vi "PH_ImageOperator.Indicate Beam Analysis.vi"(0 "i ref in":refnum<vi>, 5 "error in (no error)":errorcluster) -> (14 "i ref out":refnum<vi>, 19 "error out":errorcluster)   [LabVIEW 2014, in "PH_ImageOperator.lvlib"]
doc: "This VI sets all GUI elements related to beam anaysis."
uses:
  PH_ImageOperator.lvlib
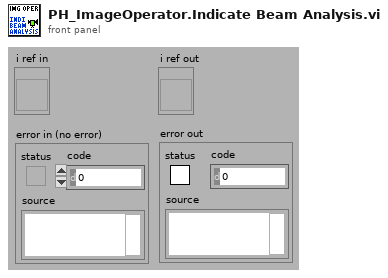
[diagram p1: front panel]
types:
  T1 = typedef "PH_ImageOperator.lvlib/PH_ImageOperator.i attribute.ctl" = cluster{"GUI Refs":cluster{"Delete":refnum<vi>, "Calibration status":refnum<vi>, "BI subtracted":refnum<vi>, "calc Energy":refnum<vi>, "Energy: expected value":refnum<vi>, "Energy: Tolerance":refnum<vi>, "Energy calculated":refnum<vi>, "Energy":refnum<vi>, "calc Beam Anal":refnum<vi>, "Maj Diam 1/esquare":refnum<vi>, "Min Diam 1/esquare":refnum<vi>, "Azi Angle":refnum<vi>, "Min/Maj Diam esquare":refnum<vi>, "Beam analysed":refnum<vi>, "CoG - x":refnum<vi>, "CoG - y":refnum<vi>, "BA: Method":refnum<vi>, "BA: Steps":refnum<vi>, "BA: Factor":refnum<vi>, "calc Traces":refnum<vi>, "Traces: Fit Gauss":refnum<vi>, "Traces calculated":refnum<vi>, "Maj FWHM":refnum<vi>, "Min FWHM":refnum<vi>, "Major Trace":refnum<vi>, "Minor Trace":refnum<vi>, "Maj Fit Order":refnum<vi>, "Min Fit Order":refnum<vi>, "Position calculated":refnum<vi>, "Position":refnum<vi>, "Type":refnum<vi>, "Center":refnum<vi>, "exp - X":refnum<vi>, "exp - Y":refnum<vi>, "Tolerance":refnum<vi>, "f":refnum<vi>, "M":refnum<vi>, "D":refnum<vi>, "q":refnum<vi>, "Dummy Method":refnum<vi>, "Dummy Type":refnum<vi>, "Global On":refnum<vi>, "Traces: No offset":refnum<vi>, "Maj 99%":refnum<vi>, "Min 99%":refnum<vi>, "GUI FF Image":refnum<vi>, "calc Fill Factor":refnum<vi>, "FF calculated":refnum<vi>, "Fill Factor: Filter?":refnum<vi>, "FF: Damage Threshold":refnum<vi>, "FF: Threshold":refnum<vi>, "FF: max allow. Energy":refnum<vi>, "FF: Fillfactor":refnum<vi>, "Calibration data":refnum<vi>}, "List of GUIs":string[], "Calibration":cluster{"Status":T2, "Calibration data":T3, "Calibration Data File":path}, "Final Image":cluster{"BI Subtraction Failure":bool}, "Energy":cluster{"on":bool, "expected value [mJ]":dbl, "Tolerance [%]":dbl, "State":T2, "Energy [mJ]":dbl, "Unit":string, "calculated @":timestamp}, "Beam Analysis":cluster{"on":bool, "Data":T4, "Method":bool, "Steps":i32, "Factor":i32, "ROI":cluster{"Left":i32, "Top":i32, "Right":i32, "Bottom":i32}, "analysed @":timestamp}, "Trace Analysis":cluster{"on":bool, "Fit on":bool, "Maj FWHM":dbl, "Min FWHM":dbl, "Maj Fit Order":i32, "Min Fit Order":i32, "No Offset":bool, "Maj 99%":dbl, "Min 99%":dbl, "Traces":cluster{"XScaleName":string, "Y Scale Minimum":sgl, "Y Scale Maximum":sgl, "X Scale Minimum":sgl, "X Scale Maximum":sgl, "Traces":cluster{"Index":sgl[], "Trace":dbl[]}[]}[], "analysed @":timestamp}, "Position Analysis":cluster{"on":bool, "exp - X":i32, "exp - Y":i32, "focal length [mm]":dbl, "Magnification":dbl, "Delta":dbl, "Theta":dbl, "Tolerance":dbl, "Type":bool, "analysed @":timestamp}, "Fill Factor":cluster{"on":bool, "Filter on?":bool, "Threshold":dbl, "Damage Threshold [J/cm²]":dbl, "Fillfactor":dbl, "Max. allowed Energy [J]":dbl, "calculated @":timestamp}, "Statistician Service ID":i32, "Images":cluster{"Background":T5, "OP":T5, "GUI":T5, "BA: ROI":T5, "Trace: Turn":T5, "FF: Main":T5, "FF: Help":T5, "PSDB: BG":T5, "PSDB: OP":T5, "PSDB: FF":T5}}
  T2 = typedef "PH_StatusHandler.lvlib/PH_StatusHandler.Status.ctl" = i16
  T3 = typedef "PH_ImageCalibrator.lvlib/PH_ImageCalibrator.Calibration Data.ctl" = cluster{"Date":string, "Time":string, "Cam Settings":cluster{"Cam ID":string, "Gain":dbl, "Brightness":dbl, "Shutter":dbl, "Cam Error":bool, "Mode":i32}, "Background Image":cluster{"Image":dbl[][], "Image Error":bool}, "Linear Calibration":cluster{"Calibration Factor":dbl, "not mm or mrad":bool}, "Energy Calibration":cluster{"Calibration Factor":dbl, "no mJ":bool}}
  T4 = typedef "PH_ImageOperator.lvlib/PH_ImageOperator.Beam Analysis Data.ctl" = cluster{"CoG-x":sgl, "CoG-y":sgl, "Maj Dim":dbl, "Min Dim":dbl, "Ellipticity":dbl, "Azimuth Angle [rad]":dbl, "Azi Angle rel to Maj?":bool}
  T5 = typedef "IMAQ Image.ctl" = refnum<image>
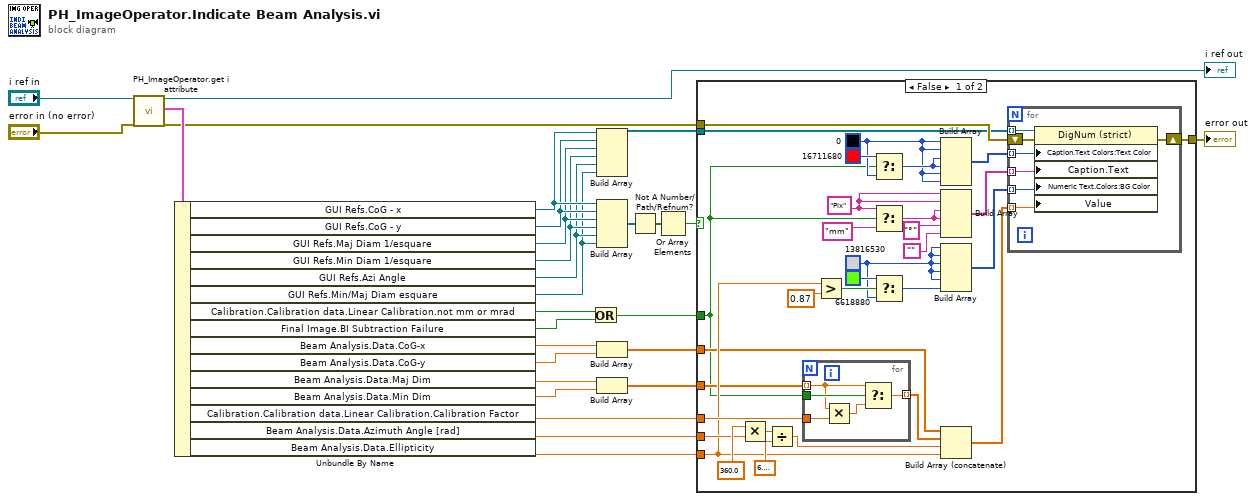
[diagram p0: block diagram]
diagram:
  n1 = call "PH_ImageOperator.get i attribute.vi"("i ref in"="i ref in", "error in (no error)"="error in (no error)") -> ("i ref out"=→"i ref out":refnum<vi>, "i attribute"=w25:T1, "error out"=w19:errorcluster)  [unwired: 15 in]
  n2 = Unbundle By Name(w25) -> ("GUI Refs.CoG - x"=w18:refnum<vi>, "GUI Refs.CoG - y"=w17:refnum<vi>, "GUI Refs.Maj Diam 1/esquare"=w16:refnum<vi>, "GUI Refs.Min Diam 1/esquare"=w15:refnum<vi>, "GUI Refs.Azi Angle"=w14:refnum<vi>, "GUI Refs.Min/Maj Diam esquare"=w13:refnum<vi>, "Calibration.Calibration data.Linear Calibration.not mm or mrad"=w3:bool, "Final Image.BI Subtraction Failure"=w2:bool, "Beam Analysis.Data.CoG-x"=w6:sgl, "Beam Analysis.Data.CoG-y"=w5:sgl, "Beam Analysis.Data.Maj Dim"=w10:dbl, "Beam Analysis.Data.Min Dim"=w11:dbl, "Calibration.Calibration data.Linear Calibration.Calibration Factor"=w8:dbl, "Beam Analysis.Data.Azimuth Angle [rad]"=w7:dbl, "Beam Analysis.Data.Ellipticity"=w12:dbl)
  n3 = Or(x=w3, y=w2) -> (x .or. y?=w1:bool)
  n4 = Build Array(w18, w17, w16, w15, w14, w13) -> (w21:refnum<vi>[])
  n5 = Build Array(w18, w17, w16, w15, w14, w13) -> (w24:refnum<vi>[])
  n6 = Build Array(w6, w5) -> (w4:sgl[])
  n7 = Build Array(w10, w11) -> (w9:dbl[])
  n8 = Not A Number/Path/Refnum?(number/path/refnum=w24) -> (NaN/Path/Refnum?=w23:bool[])
  n9 = Or Array Elements(Boolean array=w23) -> (logical OR=w22:bool)
  n10 = case shown="False" w22 {
    tunnel: w21 -> [w49 _]
    tunnel: w19 -> [w50 w72]
    tunnel: [w30 w72] -> w20
    tunnel: w12 -> [w37 _]
    tunnel: w9 -> [w31 _]
    tunnel: w8 -> [w56 _]
    tunnel: w7 -> [w52 _]
    tunnel: w4 -> [w33 _]
    tunnel: w1 -> [w29 _]
    frame False {
      w32 = u32 13816530 ("Color")
      w34 = u32 0 ("Color")
      w48 = "Pix" ("t")
      n11 = Multiply(x=360.0 ("y"), y=w52) -> (x*y=w53:dbl)
      n12 = Divide(x=w53, y=6.283185307179586) -> (x/y=w51:dbl)
      n13 = for {
        tunnel: [w64] -> w57 mode=indexing
        tunnel: w31 -> [w60] mode=indexing
        tunnel: w29 -> [w63]
        tunnel: w56 -> [w61]
        n14 = Multiply(x=w60, y=w61) -> (x*y=w62:dbl)
        n15 = Select(t=w60, s=w63, f=w62) -> (s? t:f=w64:dbl)
      }
      n16 = Greater?(x=w37, y=0.87) -> (0:w36:bool)
      n17 = Select(t=u32 16711680 ("Color"), s=w29, f=w34) -> (s? t:f=w42:u32)
      n18 = Select(t=w48, s=w29, f="mm") -> (s? t:f=w47:string)
      n19 = Select(t=u32 6618880 ("Color"), s=w36, f=w32) -> (s? t:f=w38:u32)
      n20 = Build Array(w34, w34, w42, w42, w34, w34) -> (w41:u32[])
      n21 = Build Array(w48, w48, w47, w47, "°" ("element"), "") -> (w44:string[])
      n22 = Build Array(w32, w32, w32, w32, w32, w38) -> (w40:u32[])
      n23 = Build Array (concatenate)(w33, w57, w51, w37) -> (w59:dbl[])
      n24 = for "Dig Elements" {
        tunnel: w49 -> [w69] mode=indexing
        shift-right: [w70] -> w30
        shift-left: w50 -> [w71]
        tunnel: w59 -> [w66] mode=indexing
        tunnel: w44 -> [w68] mode=indexing
        tunnel: w41 -> [w67] mode=indexing
        tunnel: w40 -> [w65] mode=indexing
        n25 = property class="DigNum (strict)"(reference=w69, error in=w71, "Caption.Text Colors:Text Color"=w67, "Caption.Text"=w68, "Numeric Text.Colors:BG Color"=w65, "Value"=w66) -> (error out=w70:errorcluster)  [unwired: 1 out]
      }
    }
    frame True {
    }
  }
  "error out" <- w20
